vi "Actor Core.vi"(8 "error in":errorcluster, 11 "Nested in":refnum<class "UI_PAPAS_USD_ING.lvclass">) -> (0 "error out":errorcluster, 3 "Actor out":refnum<class "Actor.lvclass">)   [LabVIEW 2019, in "UI_PAPAS_USD_ING.lvlib" / "UI_PAPAS_USD_ING.lvclass"]
doc: "(<B>Filename</B>: Actor Framework.lvlib:Actor.lvclass:Actor Core.vi)\n\nReceives messages to the actor, reacts to them, and initiates any error handling that may shut the actor down.\n\nDescendant classes may override this VI to append parallel tasks for the actor to complete while it handles messages. Overrides use the Call Parent Method node."
uses:
  UI_PAPAS_USD_ING.lvclass
  C:/Program Files (x86)/National Instruments/LabVIEW 2019/vi.lib/ActorFramework/Actor/Actor.lvclass
  <vilib>/ActorFramework/Actor/Actor.lvclass
  <vilib>/ActorFramework/Actor/Actor.lvclass/Actor.ctl
  <vilib>/ActorFramework/Message Enqueuer/Message Enqueuer.lvclass/Message Enqueuer.ctl
  UI_PAPAS_USD_ING.lvclass/UI_PAPAS_USD_ING.ctl
  <vilib>/ActorFramework/Message Enqueuer/Init from Existing Queue.vi
  <vilib>/ActorFramework/Message Enqueuer/Enqueue.vi
  <vilib>/ActorFramework/Stop Msg/Stop Msg.lvclass
  C:/Program Files (x86)/National Instruments/LabVIEW 2019/vi.lib/ActorFramework/Message/Message.lvclass
  <vilib>/ActorFramework/Message Priority Queue/Priority Enqueue.vi
  <vilib>/ActorFramework/Message Enqueuer/Message Enqueuer.lvclass
  BD_PAPAS_USD_ING/BD_PAPAS_USD_ING.lvclass
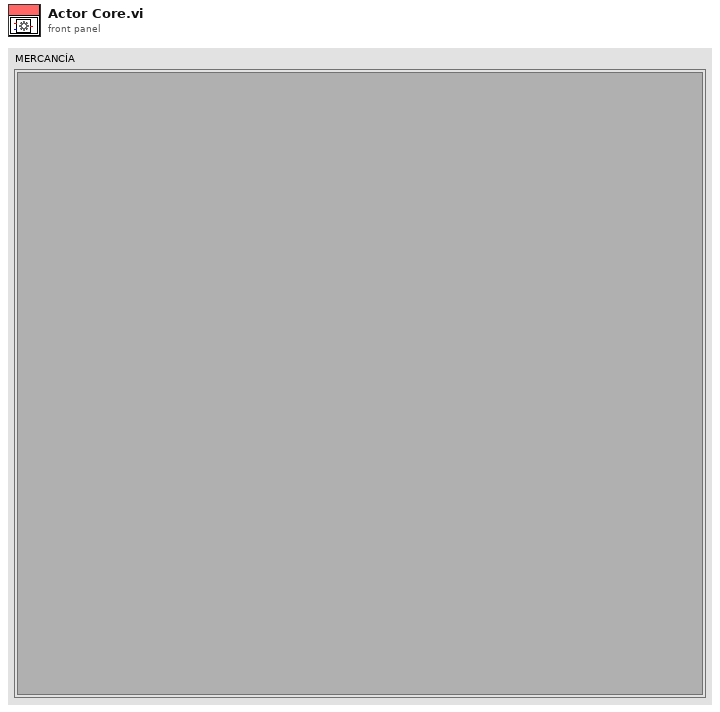
[diagram p1: front panel]
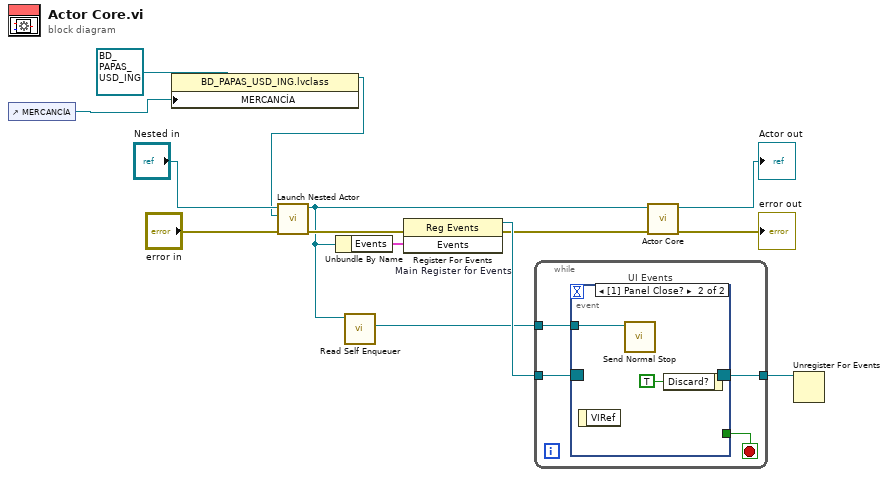
[diagram p0: block diagram]
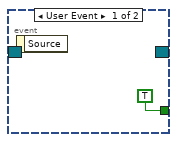
[diagram p2: hidden frame]
diagram:
  n1 = control-ref of="MERCANCÍA"() -> (w2:refnum<vi>)
  n2 = property class="BD_PAPAS_USD_ING.lvclass"(reference=refnum<class "BD_PAPAS_USD_ING.lvclass"> refnum ("BD_PAPAS_USD_ING.lvlib:BD_PAPAS_USD_ING.lvclass"), "MERCANCÍA"=w2) -> (reference out=w1:refnum<class "BD_PAPAS_USD_ING.lvclass">)  [unwired: 1 in, 1 out]
  n3 = call <vilib>:"Launch Nested Actor.vi"("error in (no error)"="error in", "Nested Actor"=w1, "Caller Actor in"="Nested in") -> ("error out"=w6:errorcluster, "Caller Actor out"=w4:refnum<class "UI_PAPAS_USD_ING.lvclass">)  [unwired: 6 in, 1 out]
  n4 = Unbundle By Name(w4) -> ("Events"=w11:cluster{"Stop":refnum<user-event>})
  n5 = call <vilib>:"Read Self Enqueuer.vi"("Actor"=w4) -> ("Self Enqueuer"=w9:refnum<class "Message Enqueuer.lvclass">)  [unwired: 10 in]
  n6 = register-events "Main Register for Events"(error in=w6, w11) -> (reference out=w12:refnum<event-registration>, error out=w7:errorcluster)  [unwired: 1 in]
  n7 = while {
    tunnel: w12 -> [w18]
    tunnel: [w16] -> w10
    tunnel: w9 -> [w15]
    stop <- w17 stop-if-true
    n8 = event "UI Events" shown="[1] Panel Close?" {
      selector: w18 -> [_ _]
      dyn-events: [_ _] -> w16
      timeout: _ -> [_ _]
      tunnel: [TRUE _] -> w17
      tunnel: w15 -> [_ w20]
      event User Event {
        n9 = event-data() -> ()  [unwired: 1 in, 1 out]
      }
      event Panel Close? {
        n10 = event-data() -> ()  [unwired: 1 in, 1 out]
        n11 = call <vilib>:"Send Normal Stop.vi"("Message Enqueuer"=w20) -> ()  [unwired: 10 in, 1 out]
        n12 = event-data("Discard?"=TRUE) -> ()  [unwired: 1 in, 1 out]
      }
    }
  }
  n13 = call-parent "Actor Core.vi"("error in"=w7, "Actor in"=w4) -> ("error out"=→"error out":errorcluster, "Actor out"=→"Actor out":refnum<class "Actor.lvclass">)  [unwired: 8 in]
  n14 = Unregister For Events(event registration refnum=w10) -> ()  [unwired: 1 in, 1 out]
